vi "Read Challenge Data.vi"(8 "error in (no error)":errorcluster) -> (0 "error out":errorcluster, 3 "Word List":string[](array[string]))   [LabVIEW 2024, in "Wordle Scorer.lvlib"]
uses:
  Wordle Scorer.lvlib
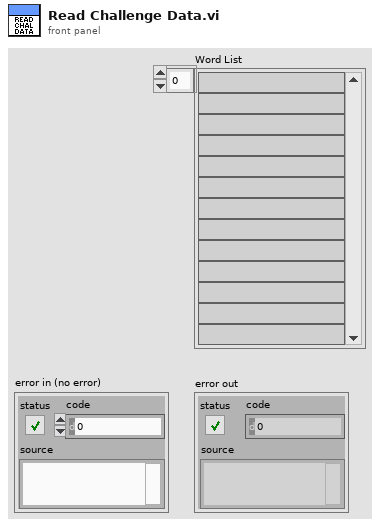
[diagram p1: front panel]
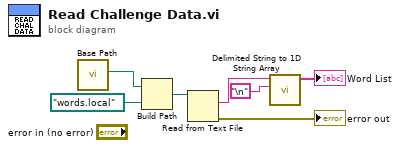
[diagram p0: block diagram]
diagram:
  n1 = call "Base Path.vi"() -> ("Base Path"=w7:path)  [unwired: 11 in]
  n2 = Build Path(base path=w7, name or relative path=path "words.local") -> (appended path=w5:path)
  n3 = Read from Text File(file (use dialog)=w5) -> (text=w3:string, error out=→"error out":errorcluster)  [unwired: 3 in, 2 out]
  n4 = call <vilib>:"Delimited String to 1D String Array.vi"("delimiter"="\n", "delimited string"=w3) -> ("string array"=→"Word List":string[])  [unwired: 9 in]
